vi "ASDA-A2_Motor Home Setting.vi"(8 "error in":errorcluster, 10 "Motor Home Setting":T1={"Reach Limit"=enum."Return", "Z Phase"=enum."Return", "Direction"=enum."Negative", "First High Speed(0.1RPM)"=1000, "Second Low Speed(0.1RPM)"=200, "Home Position"=0}, 11 "Buffer Data In":T2) -> (0 "error out":errorcluster, 3 "Buffer Data Out":T2)   [LabVIEW 2016]
uses:
  Data Def/ASDA-A2_Buffer Data.ctl
  Data Def/ASDA-A2_Write Register Data.ctl
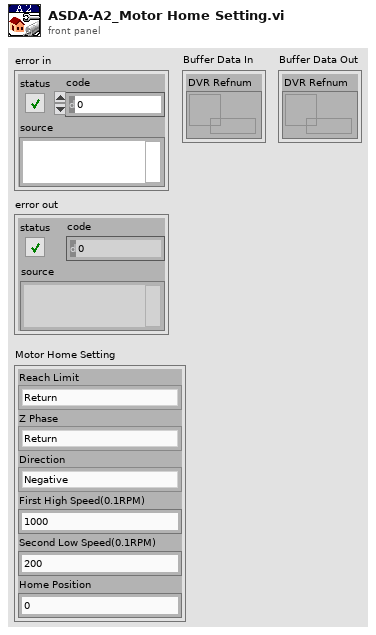
[diagram p1: front panel]
types:
  T1 = cluster{"Reach Limit":enum8{"Alarm", "Return"}, "Z Phase":enum8{"Return", "Forward", "Ignore"}, "Direction":enum8{"Position", "Negative", "Position+DI OFF->ON  Limit", "Negative+DI OFF->ON Limit", "Position+Find Z", "Negative+Find Z", "Position+DI ON->OFF  Limit", "Negative+DI ON->OFF  Limit", "Location ORG", "Position+DI Limit", "Negative+DI Limit"}, "First High Speed(0.1RPM)":u32, "Second Low Speed(0.1RPM)":u32, "Home Position":i32}
  T2 = typedef "ASDA-A2_Buffer Data.ctl" = cluster{"DVR Refnum":refnum<data-value>}
  T3 = typedef "ASDA-A2_Write Register Data.ctl" = cluster{"Address":u16, "Max Value":u32, "Min Value":u32, "Value":u32, "Type":enum16{"16 Bits", "32 Bits"}, "Page":string, "Description":string}
  T4 = enum8{"Position", "Negative", "Position+DI OFF->ON  Limit", "Negative+DI OFF->ON Limit", "Position+Find Z", "Negative+Find Z", "Position+DI ON->OFF  Limit", "Negative+DI ON->OFF  Limit", "Location ORG", "Position+DI Limit", "Negative+DI Limit"}
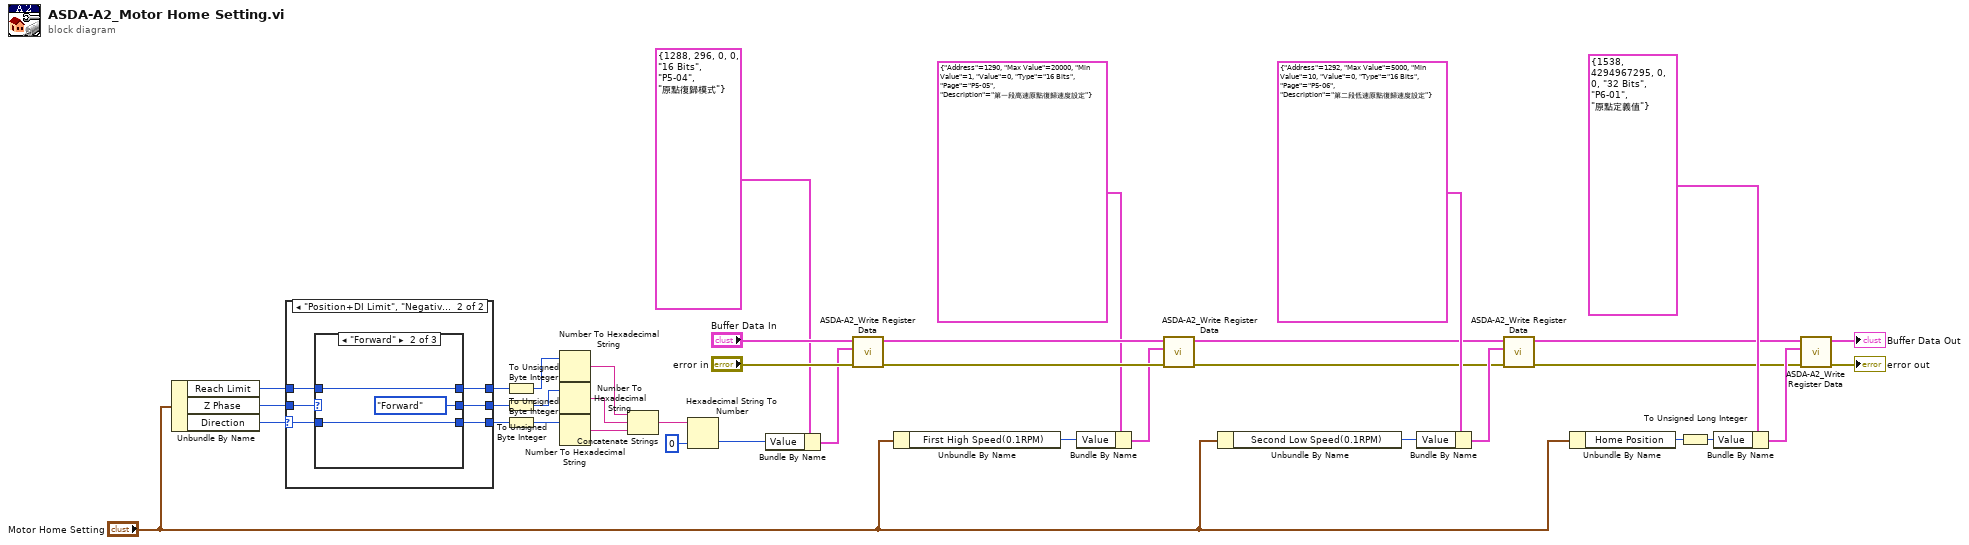
[diagram p0: block diagram]
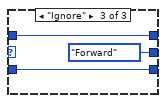
[diagram p4: hidden frame]
diagram:
  n1 = Unbundle By Name("Motor Home Setting") -> ("Reach Limit"=w4:enum8{"Alarm", "Return"}, "Z Phase"=w5:enum8{"Return", "Forward", "Ignore"}, "Direction"=w6:T4)
  n2 = case shown="\"Position+DI Limit\", \"Negative+DI Limit\"" w6 {
    selector: w6 -> [w39 w44]
    tunnel: w5 -> [w40 w47]
    tunnel: w4 -> [w41 w46]
    tunnel: [w41 w45] -> w3
    tunnel: [w40 w42] -> w2
    tunnel: [w39 w43] -> w1
    frame "Position", Default {
    }
    frame "Position+DI Limit", "Negative+DI Limit" {
      n3 = case shown="\"Forward\"" w47 {
        selector: w47 -> [w49 _ _]
        tunnel: w46 -> [w50 w53 w56]
        tunnel: [w50 w53 w56] -> w45
        tunnel: w44 -> [w48 w52 w54]
        tunnel: [w48 w52 w54] -> w43
        tunnel: [w49 enum8{"Return", "Forward", "Ignore"}."Forward" ("Z Phase") enum8{"Return", "Forward", "Ignore"}."Forward" ("Z Phase")] -> w42
        frame "Return", Default {
        }
        frame "Forward" {
        }
        frame "Ignore" {
        }
      }
    }
  }
  n4 = To Unsigned Byte Integer(number=w3) -> (unsigned 8bit integer=w33:u8)
  n5 = To Unsigned Byte Integer(number=w2) -> (unsigned 8bit integer=w34:u8)
  n6 = To Unsigned Byte Integer(number=w1) -> (unsigned 8bit integer=w35:u8)
  n7 = Number To Hexadecimal String(2:w33) -> (0:w30:string)  [unwired: 1 in]
  n8 = Number To Hexadecimal String(2:w34) -> (0:w31:string)  [unwired: 1 in]
  n9 = Number To Hexadecimal String(2:w35) -> (0:w32:string)  [unwired: 1 in]
  n10 = Concatenate Strings(w30, w31, w32) -> (w29:string)
  n11 = Hexadecimal String To Number(string=w29, default (0uL)=u32 0 ("default (0 U32)")) -> (number=w7:u32)  [unwired: 1 in, 1 out]
  n12 = Bundle By Name(cluster=T3 {"Address"=1288, "Max Value"=296, "Min Value"=0, "Value"=0, "Type"=enum."16 Bits", "Page"="P5-04", "Description"="原點復歸模式"} ("Write Register Data"), "Value"=w7) -> (w24:T3)
  n13 = call "ASDA-A2_Write Register Data.vi"("error in"="error in", "Write Register Data"=w24, "Buffer Data In"="Buffer Data In") -> ("error out"=w23:errorcluster, "Buffer Data Out"=w22:T2)  [unwired: 7 in]
  n14 = Unbundle By Name("Motor Home Setting") -> ("First High Speed(0.1RPM)"=w20:u32)
  n15 = Bundle By Name(cluster=T3 {"Address"=1290, "Max Value"=20000, "Min Value"=1, "Value"=0, "Type"=enum."16 Bits", "Page"="P5-05", "Description"="第一段高速原點復歸速度設定"} ("Write Register Data"), "Value"=w20) -> (w19:T3)
  n16 = call "ASDA-A2_Write Register Data.vi"("error in"=w23, "Write Register Data"=w19, "Buffer Data In"=w22) -> ("error out"=w14:errorcluster, "Buffer Data Out"=w15:T2)  [unwired: 7 in]
  n17 = Unbundle By Name("Motor Home Setting") -> ("Second Low Speed(0.1RPM)"=w17:u32)
  n18 = Bundle By Name(cluster=T3 {"Address"=1292, "Max Value"=5000, "Min Value"=10, "Value"=0, "Type"=enum."16 Bits", "Page"="P5-06", "Description"="第二段低速原點復歸速度設定"} ("Write Register Data"), "Value"=w17) -> (w18:T3)
  n19 = call "ASDA-A2_Write Register Data.vi"("error in"=w14, "Write Register Data"=w18, "Buffer Data In"=w15) -> ("error out"=w10:errorcluster, "Buffer Data Out"=w11:T2)  [unwired: 7 in]
  n20 = Unbundle By Name("Motor Home Setting") -> ("Home Position"=w9:i32)
  n21 = To Unsigned Long Integer(number=w9) -> (unsigned 32bit integer=w8:u32)
  n22 = Bundle By Name(cluster=T3 {"Address"=1538, "Max Value"=4294967295, "Min Value"=0, "Value"=0, "Type"=enum."32 Bits", "Page"="P6-01", "Description"="原點定義值"} ("Write Register Data"), "Value"=w8) -> (w12:T3)
  n23 = call "ASDA-A2_Write Register Data.vi"("error in"=w10, "Write Register Data"=w12, "Buffer Data In"=w11) -> ("error out"=→"error out":errorcluster, "Buffer Data Out"=→"Buffer Data Out":T2)  [unwired: 7 in]
